vi "HV Full Monitor Live.vi"(11 "stop":bool) -> (3 "Monitor Cluster Live":T1)   [LabVIEW 2018, in "HV QMH.lvlib"]
uses:
  HV QMH.lvlib
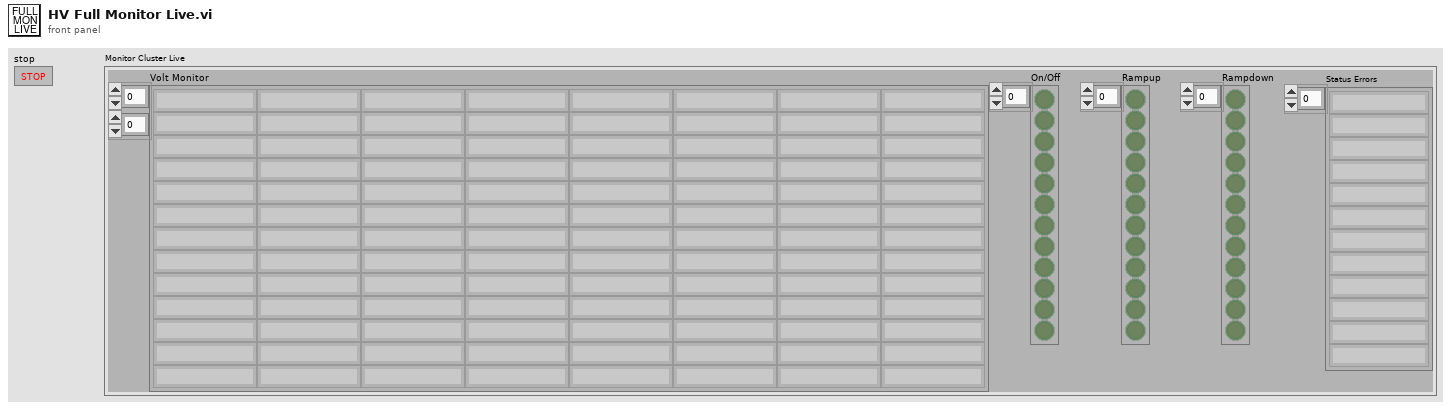
[diagram p1: front panel]
types:
  T1 = cluster{"Volt Monitor":string[][], "On/Off":bool[], "Rampup":bool[], "Rampdown":bool[], "Status Errors":string[]}
  T2 = cluster{"Monitor":string[][], "On/Off":bool[], "Rampup":bool[], "Rampdown":bool[], "Status Errors":string[]}
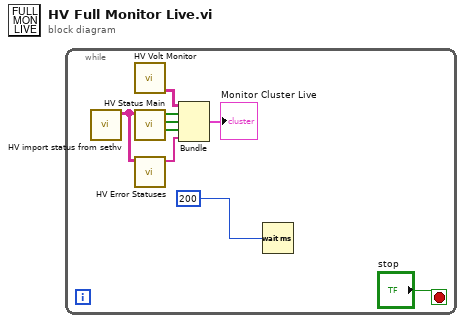
[diagram p0: block diagram]
diagram:
  n1 = while {
    stop <- "stop" stop-if-true
    n2 = call "HV import status from sethv.vi"() -> ("transposed array"=w9:string[][])  [unwired: 10 in, 1 out]
    n3 = call "HV Volt Monitor.vi"() -> ("Monitor"=w8:string[][])  [unwired: 11 in]
    n4 = call "HV Status Main.vi"("Status Array"=w9) -> ("Rampdown"=w5:bool[], "Rampup"=w6:bool[], "On/Off"=w7:bool[])  [unwired: 8 in]
    n5 = call "HV Error Statuses.vi"("transposed array"=w9) -> ("Status Errors"=w4:string[])  [unwired: 10 in]
    n6 = Bundle("Monitor"=w8, "On/Off"=w7, "Rampup"=w6, "Rampdown"=w5, "Status Errors"=w4) -> (→"Monitor Cluster Live":T2)  [unwired: 1 in]
    n7 = Wait (ms)(milliseconds to wait=u32 200) -> ()  [unwired: 1 out]
  }
